vi "Altitude Conttrol.vi"(7 "Stop":bool, 11 "AltLim":cluster{"Max":dbl, "Min":dbl}) -> (3 "AltSP":i32)   [LabVIEW 2013]
uses:
  Type Defs/Alt Control.ctl
  Type Defs/Alt Digit 100 New.ctl
panel:
  in  "Confirm Now":bool
  in  "ALT SET":T1 {"Alt Digit 100" min=0 max=9 step=1; "Alt Digit 100" min=0 max=9 step=1; "Alt Digit 100" min=0 max=9 step=1; "Alt Digit 100" min=0 max=9 step=1; "Alt Digit 100" min=0 max=9 step=1}
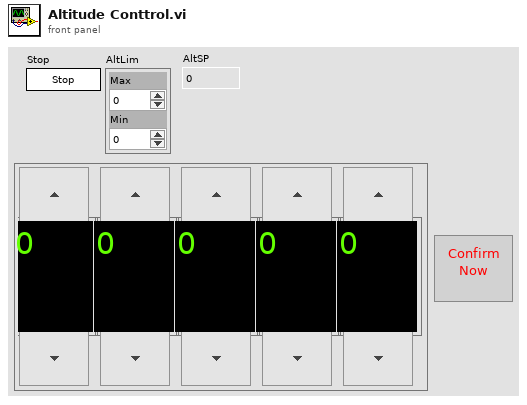
[diagram p1: front panel]
types:
  T1 = typedef "Alt Control.ctl" = cluster{"Alt Digit 100":T2, "Alt Digit 100":T2, "Alt Digit 100":T2, "Alt Digit 100":T2, "Alt Digit 100":T2}
  T2 = typedef "Alt Digit 100 New.ctl" = i8
  T3 = cluster{"[0]":i8, "[1]":i8, "[2]":i8, "[3]":i8, "[4]":i8}
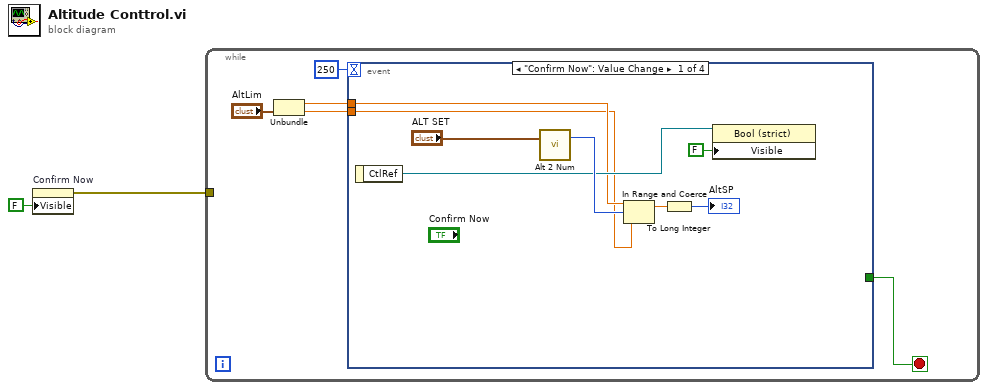
[diagram p0: block diagram]
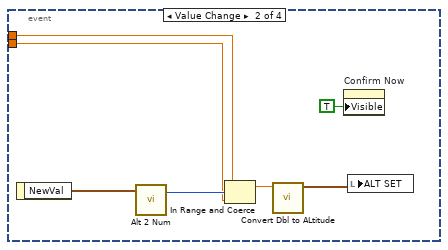
[diagram p2: hidden frame]
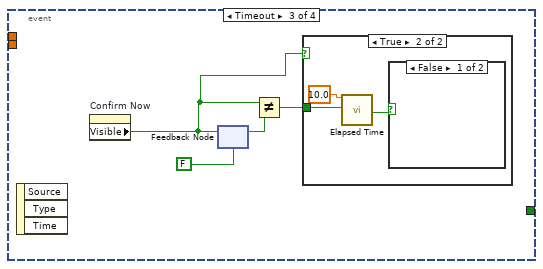
[diagram p3: hidden frame]
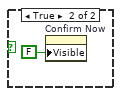
[diagram p5: hidden frame]
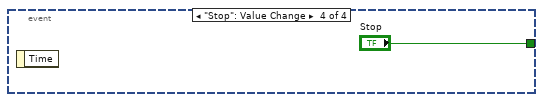
[diagram p6: hidden frame]
diagram:
  n1 = property on="Confirm Now" class="Bool (strict)"("Visible"=FALSE) -> (error out=w1:errorcluster)  [unwired: 2 in, 1 out]
  n2 = while {
    tunnel: w1 -> [_]
    stop <- w4 stop-if-true
    n3 = Unbundle("AltLim") -> ("Max"=w6:dbl, "Min"=w5:dbl)
    n4 = event shown="[0] \"Confirm Now\": Value Change" {
      selector: _ -> [_ _ _ _]
      dyn-events: _ -> [_ _ _ _]
      timeout: 250 -> [_ _ _ _]
      tunnel: w6 -> [w9 w18 _ _]
      tunnel: w5 -> [w8 w17 _ _]
      tunnel: [_ _ _ "Stop"] -> w4
      event "Confirm Now": Value Change {
        n5 = event-data() -> ("CtlRef"=w11:refnum<vi>)  [unwired: 1 in]
        n6 = call "Alt 2 Num.vi"("Alt Ctl"="ALT SET") -> ("Alt"=w15:i32)  [unwired: 2 in]
        n7 = In Range and Coerce(upper limit=w9, x=w15, lower limit=w8) -> (coerced(x)=w13:dbl)  [unwired: 1 out]
        n8 = To Long Integer(number=w13) -> (32bit integer=→"AltSP":i32)
        n9 = property class="Bool (strict)"(reference=w11, "Visible"=FALSE) -> ()  [unwired: 1 in, 2 out]
      }
      event Value Change {
        n10 = event-data() -> ("NewVal"=w19:T1)  [unwired: 1 in]
        n11 = call "Alt 2 Num.vi"("Alt Ctl"=w19) -> ("Alt"=w21:i32)  [unwired: 2 in]
        n12 = In Range and Coerce(upper limit=w18, x=w21, lower limit=w17) -> (coerced(x)=w20:dbl)  [unwired: 1 out]
        n13 = call "Convert Dbl to ALtitude.vi"("Setpoint"=w20) -> ("Altitude Out"=w16:T3)  [unwired: 10 in]
        n14 = property on="Confirm Now" class="Bool (strict)"("Visible"=TRUE) -> ()  [unwired: 2 in, 2 out]
        n15 = local write "ALT SET"(w16) -> ()
      }
      event Timeout {
        n16 = event-data() -> ()  [unwired: 1 in, 3 out]
        n17 = property on="Confirm Now" class="Bool (strict)"() -> ("Visible"=w24:bool)  [unwired: 2 in, 2 out]
        n18 = feedback-in #1(w24) -> ()
        n19 = feedback #1(FALSE ("Visible")) -> (w25:bool)
        n20 = Not Equal?(x=w24, y=w25) -> (x != y?=w23:bool)
        n21 = case shown="True" w24 {
          tunnel: w23 -> [_ w28]
          frame False {
          }
          frame True {
            n22 = call "Elapsed Time"("Time Target (s)"=10.0, "Reset"=w28) -> ("Time has Elapsed"=w27:bool)  [unwired: 10 in, 7 out]
            n23 = case shown="False" w27 {
              frame False {
              }
              frame True {
                n24 = property on="Confirm Now" class="Bool (strict)"("Visible"=FALSE) -> ()  [unwired: 2 in, 2 out]
              }
            }
          }
        }
      }
      event "Stop": Value Change {
        n25 = event-data() -> ()  [unwired: 1 in, 1 out]
      }
    }
  }
